vi "VScaleInfo.vi"   [LabVIEW 2022 SP3]
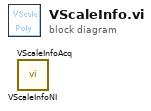
[diagram p0: block diagram]
diagram:
  n1 = call "VScaleInfoNI.vi"() -> ()  [unwired: 7 in, 4 out]
  n2 = call "VScaleInfoAcq.vi"() -> ()  [unwired: 7 in, 4 out]
